vi "空调控制.vi"() -> ()   [LabVIEW 2016, in "环境动力监测库.lvlib" / "空调库.lvlib"]
uses:
  <vilib>/Utility/miscctls.llb/LVPointTypeDef.ctl
panel:
  in  "变更空调型号":bool
  out "布尔":bool
  # "空调监测"
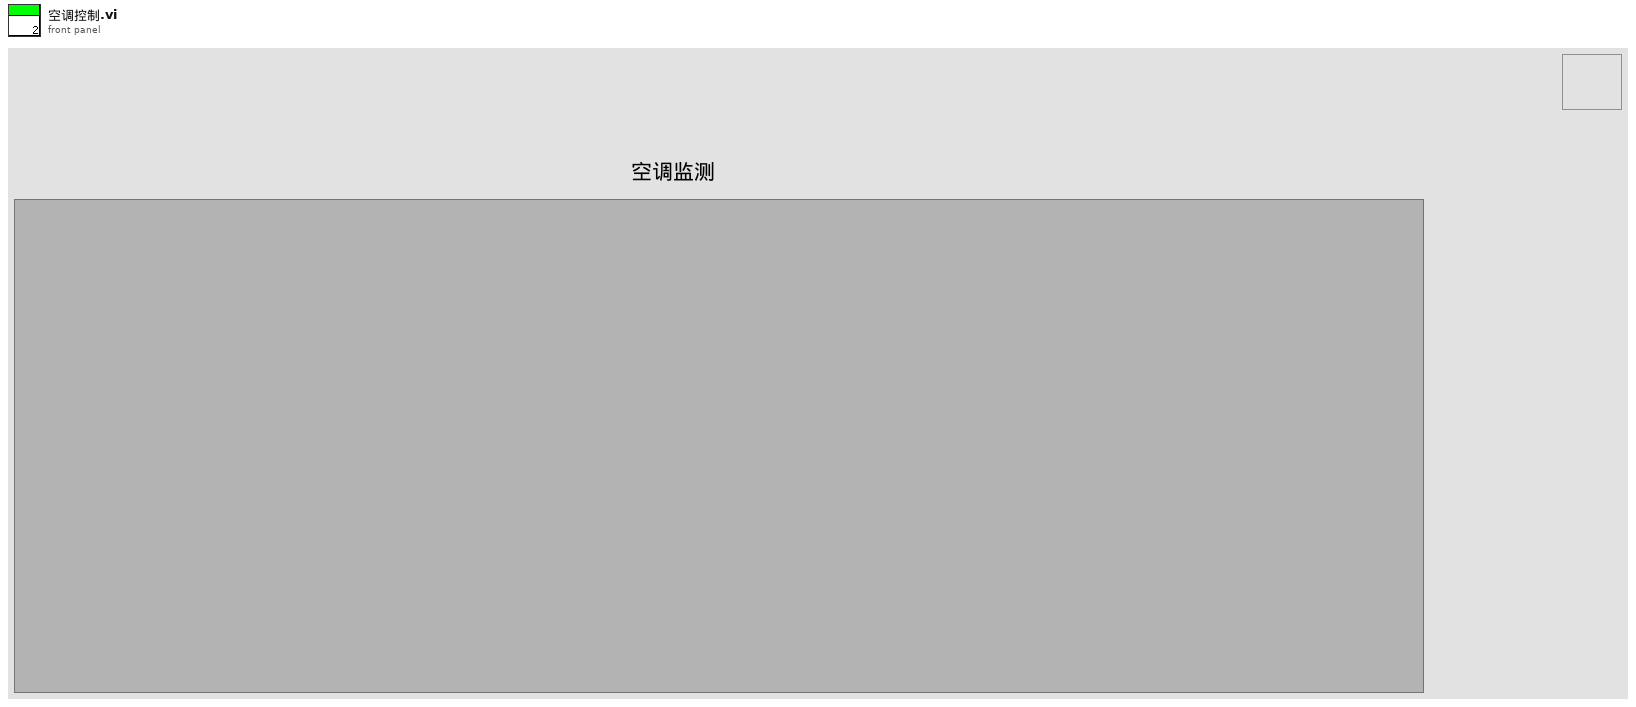
[diagram p1: front panel]
types:
  T1 = typedef "LVPointTypeDef.ctl" = cluster{"Horizontal":i16, "Vertical":i16}
  T2 = cluster{"型号选择":enum16{"黑盾", "英维克", "仁科测控RS-KTC-N01"}, "MB session in":refnum<class "MB_Master.lvclass">, "英维克空调寄存器":u16[], "通讯状态":bool, "PORT":string, "IP":string, "Slave ID ":u8, "Serial Config":cluster{"baud rate (bps)":u32, "stop bits":u16, "parity":u16, "flow control":u16, "timeout":u32, "retries":i32}, "VISA Resource":refnum<visa-resource-name>, "MB通信方式选择":enum16{"串口", "TCP"}, "系统参数":cluster{"空调开启点":u16, "空调灵敏点":u16, "加热开启点":u16, "加热灵敏度":u16, "高温告警点":u16, "低温告警点":u16}}
  T3 = enum32{"Bad", "Idle", "Run top level", "Running"}
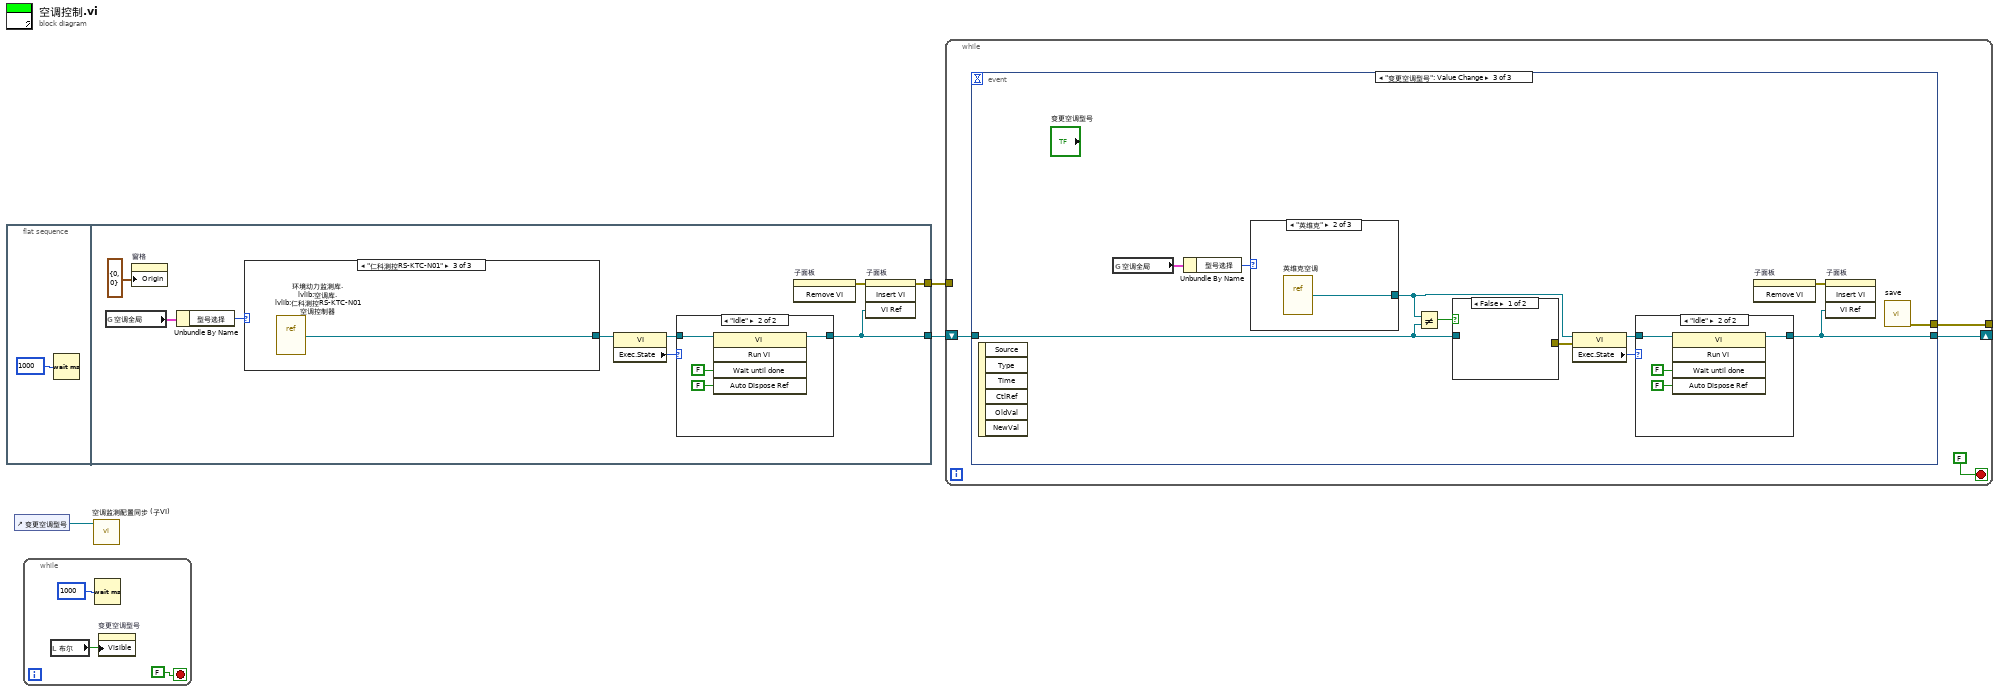
[diagram p0: block diagram]
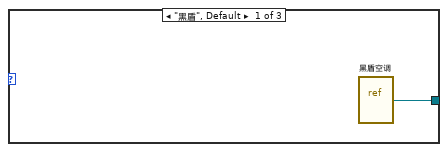
[diagram p2: hidden frame]
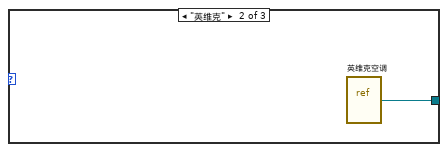
[diagram p3: hidden frame]
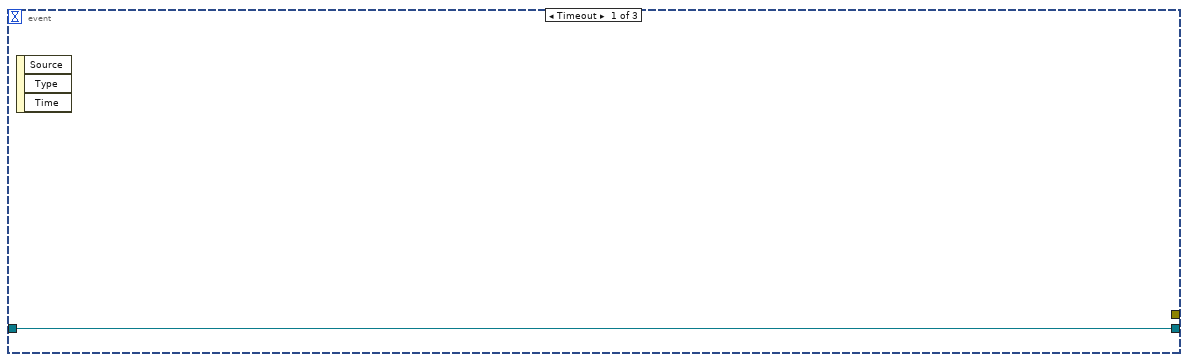
[diagram p5: hidden frame]
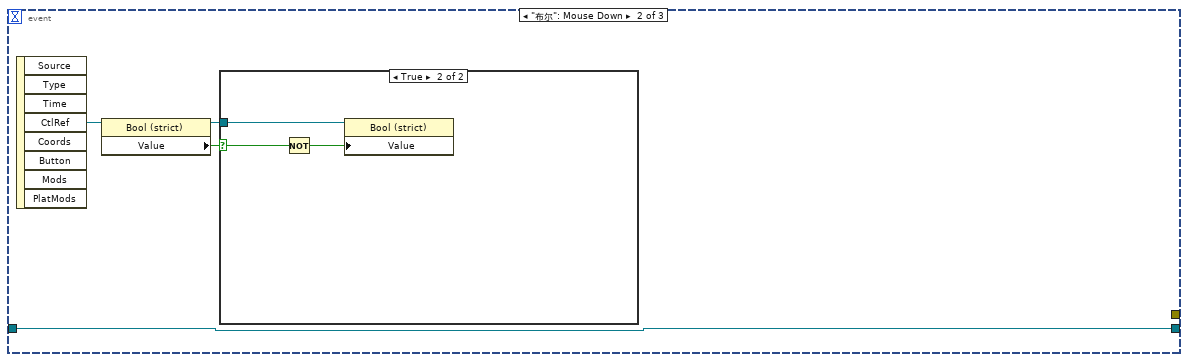
[diagram p6: hidden frame]
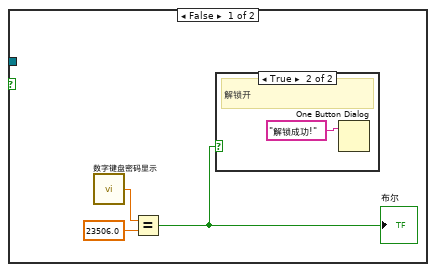
[diagram p7: hidden frame]
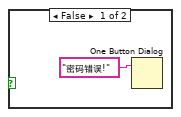
[diagram p8: hidden frame]
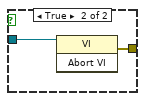
[diagram p9: hidden frame]
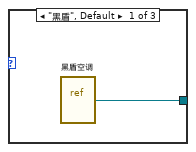
[diagram p10: hidden frame]
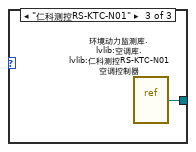
[diagram p11: hidden frame]
diagram:
  n1 = flat-sequence {
    tunnel: [w10] -> w3
    tunnel: [w9] -> w2
    frame #0 {
      n2 = Wait (ms)(milliseconds to wait=u32 1000 ("等待时间（毫秒）")) -> ()  [unwired: 1 out]
    }
    frame #1 {
      n3 = global read "断电保存全局变量.vi" "空调全局"() -> (w6:T2)
      n4 = property on="窗格" class="Pane"("Origin"=T1 {"Horizontal"=0, "Vertical"=0} ("原点")) -> ()  [unwired: 2 in, 2 out]
      n5 = Unbundle By Name(w6) -> ("型号选择"=w5:enum16{"黑盾", "英维克", "仁科测控RS-KTC-N01"})
      n6 = case shown="\"仁科测控RS-KTC-N01\"" w5 {
        tunnel: [w14 w15 w16] -> w7
        frame "黑盾", Default {
          n7 = vi-ref "黑盾空调.vi"() -> (w14:refnum<vi>)
        }
        frame "英维克" {
          n8 = vi-ref "英维克空调.vi"() -> (w15:refnum<vi>)
        }
        frame "仁科测控RS-KTC-N01" {
          n9 = vi-ref "环境动力监测库.lvlib:空调库.lvlib:仁科测控RS-KTC-N01空调控制器.vi"() -> (w16:refnum<vi>)
        }
      }
      n10 = property class="VI"(reference=w7) -> (reference out=w12:refnum<vi>, "Exec.State"=w13:T3)  [unwired: 1 in, 1 out]
      n11 = case shown="\"Idle\"" w13 {
        tunnel: w12 -> [w17 w19]
        tunnel: [w17 w18] -> w9
        frame "Bad", Default {
        }
        frame "Idle" {
          n12 = invoke class="VI" method="Run VI"(reference=w19, "Wait until done"=FALSE ("结束前等待"), "Auto Dispose Ref"=FALSE ("自动销毁引用")) -> (reference out=w18:refnum<vi>)  [unwired: 2 in, 4 out]
        }
      }
      n13 = invoke on="子面板" class="SubPnl" method="Remove VI"() -> (error out=w11:errorcluster)  [unwired: 3 in, 2 out]
      n14 = invoke on="子面板" class="SubPnl" method="Insert VI"(error in=w11, "VI Ref"=w9) -> (error out=w10:errorcluster)  [unwired: 2 in, 3 out]
    }
  }
  n15 = control-ref of="变更空调型号"() -> (w1:refnum<vi>)
  n16 = while {
    stop <- FALSE stop-if-true
    n17 = local read "布尔"() -> (w23:bool)
    n18 = Wait (ms)(milliseconds to wait=u32 1000 ("等待时间（毫秒）")) -> ()  [unwired: 1 out]
    n19 = property on="变更空调型号" class="Bool (strict)"("Visible"=w23) -> ()  [unwired: 2 in, 2 out]
  }
  n20 = call "空调监测配置同步 (子VI).vi"("Boolean输入"=w1) -> ()  [unwired: 11 in]
  n21 = while {
    tunnel: w3 -> [_]
    tunnel: [w28] -> _
    shift-right: [w27] -> _
    shift-left: w2 -> [w26]
    stop <- FALSE stop-if-true
    n22 = event shown="[2] \"变更空调型号\": Value Change" {
      selector: _ -> [_ _ _]
      dyn-events: _ -> [_ _ _]
      timeout: _ -> [_ _ _]
      tunnel: [_ _ w44] -> w28
      tunnel: [w29 w30 w52] -> w27
      tunnel: w26 -> [w29 w30 w47]
      event Timeout {
        n23 = event-data() -> ()  [unwired: 1 in, 3 out]
      }
      event "布尔": Mouse Down {
        n24 = event-data() -> ("CtlRef"=w33:refnum<vi>)  [unwired: 1 in, 7 out]
        n25 = property class="Bool (strict)"(reference=w33) -> (reference out=w31:refnum<vi>, "Value"=w32:bool)  [unwired: 1 in, 1 out]
        n26 = case shown="True" w32 {
          selector: w32 -> [_ w41]
          tunnel: w31 -> [_ w40]
          frame False {
            n27 = call "数字键盘密码显示.vi"() -> ("NewNumber"=w36:sgl)  [unwired: 1 in]
            n28 = Equal?(x=w36, y=sgl 23506.0) -> (x = y?=w34:bool)
            "布尔" <- w34
            n29 = case shown="True" w34 {
              frame False {
                n30 = One Button Dialog(message="密码错误!" ("消息")) -> ()  [unwired: 1 in, 1 out]
              }
              frame True {
                # "解锁开"
                n31 = One Button Dialog(message="解锁成功!" ("消息")) -> ()  [unwired: 1 in, 1 out]
              }
            }
          }
          frame True {
            n32 = Not(x=w41) -> (.not. x?=w39:bool)
            n33 = property class="Bool (strict)"(reference=w40, "Value"=w39) -> ()  [unwired: 1 in, 2 out]
          }
        }
      }
      event "变更空调型号": Value Change {
        n34 = event-data() -> ()  [unwired: 1 in, 6 out]
        n35 = global read "断电保存全局变量.vi" "空调全局"() -> (w43:T2)
        n36 = Unbundle By Name(w43) -> ("型号选择"=w42:enum16{"黑盾", "英维克", "仁科测控RS-KTC-N01"})
        n37 = case shown="\"英维克\"" w42 {
          tunnel: [w55 w56 w57] -> w46
          frame "黑盾", Default {
            n38 = vi-ref "黑盾空调.vi"() -> (w55:refnum<vi>)
          }
          frame "英维克" {
            n39 = vi-ref "英维克空调.vi"() -> (w56:refnum<vi>)
          }
          frame "仁科测控RS-KTC-N01" {
            n40 = vi-ref "环境动力监测库.lvlib:空调库.lvlib:仁科测控RS-KTC-N01空调控制器.vi"() -> (w57:refnum<vi>)
          }
        }
        n41 = Not Equal?(x=w46, y=w47) -> (x != y?=w45:bool)
        n42 = case shown="False" w45 {
          tunnel: w47 -> [_ w54]
          tunnel: [_ w53] -> w48
          frame False {
          }
          frame True {
            n43 = invoke class="VI" method="Abort VI"(reference=w54) -> (error out=w53:errorcluster)  [unwired: 2 in, 2 out]
          }
        }
        n44 = property class="VI"(reference=w46, error in=w48) -> (reference out=w50:refnum<vi>, "Exec.State"=w51:T3)  [unwired: 1 out]
        n45 = case shown="\"Idle\"" w51 {
          tunnel: w50 -> [w58 w60]
          tunnel: [w58 w59] -> w52
          frame "Bad", Default {
          }
          frame "Idle" {
            n46 = invoke class="VI" method="Run VI"(reference=w60, "Wait until done"=FALSE ("结束前等待"), "Auto Dispose Ref"=FALSE ("自动销毁引用")) -> (reference out=w59:refnum<vi>)  [unwired: 2 in, 4 out]
          }
        }
        n47 = invoke on="子面板" class="SubPnl" method="Remove VI"() -> (error out=w49:errorcluster)  [unwired: 3 in, 2 out]
        n48 = invoke on="子面板" class="SubPnl" method="Insert VI"(error in=w49, "VI Ref"=w52) -> ()  [unwired: 2 in, 4 out]
        n49 = call "save.vi"() -> ("error out"=w44:errorcluster)  [unwired: 11 in]
      }
    }
  }
